vi "StringDateTimeMinusNow.vi"(10 "String DateTime":string) -> (2 "DateTime - Now":dbl format="%#.2f")   [LabVIEW 2012]
uses:
  <vilib>/Utility/miscctls.llb/LVDateTimeRec.ctl
panel:
  in  "date time rec":T1
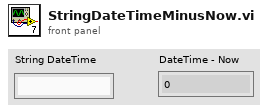
[diagram p1: front panel]
types:
  T1 = typedef "LVDateTimeRec.ctl" = cluster{"fractional second":dbl, "second":i32, "minute":i32, "hour":i32, "day of month":i32, "month":i32, "year":i32, "day of week":i32, "day of year":i32, "DST":i32}
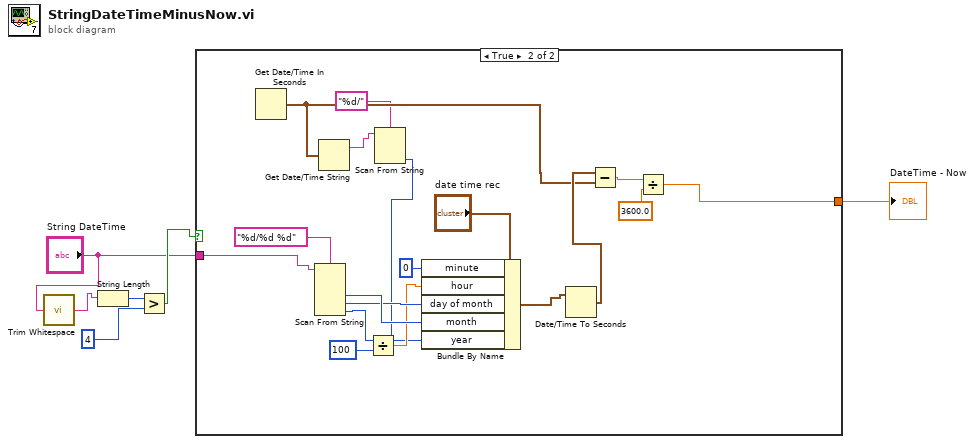
[diagram p0: block diagram]
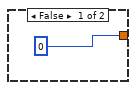
[diagram p2: hidden frame]
diagram:
  n1 = call <vilib>:"Trim Whitespace.vi"("string"="String DateTime") -> ("trimmed string"=w1:string)  [unwired: 1 in]
  n2 = String Length(string=w1) -> (length=w6:i32)
  n3 = Greater?(x=w6, y=4) -> (0:w4:bool)
  n4 = case shown="True" w4 {
    tunnel: "String DateTime" -> [_ w9]
    tunnel: [0 w8] -> w3
    frame False {
    }
    frame True {
      n5 = Get Date/Time In Seconds() -> (seconds since 1Jan1904=w13:timestamp)
      n6 = Scan From String(format string="%d/%d %d", input string=w9) -> (output 1=w23:i32, output 2=w22:i32, output 3=w21:i32)  [unwired: 5 in, 3 out]
      n7 = Get Date/Time String(seconds (now)=w13) -> (date string=w12:string)  [unwired: 2 in, 1 out]
      n8 = Divide(x=w21, y=100) -> (x/y=w19:dbl)
      n9 = Scan From String(format string="%d/", input string=w12) -> (output 1=w10:i32)  [unwired: 3 in, 3 out]
      n10 = Bundle By Name(cluster="date time rec", "minute"=0, "hour"=w19, "day of month"=w22, "month"=w23, "year"=w10) -> (w17:T1)
      n11 = Date/Time To Seconds(2:w17) -> (0:w14:timestamp)  [unwired: 1 in]
      n12 = Subtract(x=w14, y=w13) -> (x-y=w16:dbl)
      n13 = Divide(x=w16, y=3600.0) -> (x/y=w8:dbl)
    }
  }
  "DateTime - Now" <- w3
